vi "Actor Core.vi"(8 "error in":errorcluster, 11 "Nested in":refnum<class "ActorUITemplate.lvclass">) -> (0 "error out":errorcluster, 3 "Actor out":refnum<class "Actor.lvclass">)   [LabVIEW 2021, in "ActorUITemplate.lvclass"]
doc: "(<B>Filename</B>: Actor Framework.lvlib:Actor.lvclass:Actor Core.vi)\n\nReceives messages to the actor, reacts to them, and initiates any error handling that may shut the actor down.\n\nDescendant classes may override this VI to append parallel tasks for the actor to complete while it handles messages. Overrides use the Call Parent Method node."
uses:
  ActorUITemplate.lvclass
  C:/Program Files (x86)/National Instruments/LabVIEW 2021/user.lib/John_Lib/AbstractActorTemplate/AbstractActorTemplate/UIActorTop.lvclass
  C:/Program Files (x86)/National Instruments/LabVIEW 2021/vi.lib/ActorFramework/Actor/Actor.lvclass
  <vilib>/ActorFramework/Actor/Actor.lvclass
  TopRef.ctl
  ActorUITemplate.lvclass/ActorUITemplate.ctl
  <vilib>/ActorFramework/Actor/Actor.lvclass/Actor.ctl
  <vilib>/ActorFramework/Message Enqueuer/Message Enqueuer.lvclass/Message Enqueuer.ctl
  <vilib>/ActorFramework/Message Enqueuer/Init from Existing Queue.vi
  <vilib>/ActorFramework/Message Enqueuer/Enqueue.vi
  <vilib>/ActorFramework/Stop Msg/Stop Msg.lvclass
  C:/Program Files (x86)/National Instruments/LabVIEW 2021/vi.lib/ActorFramework/Message/Message.lvclass
  <vilib>/Utility/error.llb/Trim Whitespace.vi
  <vilib>/ActorFramework/Message Priority Queue/Priority Enqueue.vi
  <userlib>/John_Lib/OPCUA/OPCUA.lvclass
  <vilib>/ActorFramework/Message Enqueuer/Message Enqueuer.lvclass
  <userlib>/John_Lib/AbstractActorTemplate/AbstractActorTemplate/UIActorTop.lvclass
  C:/Program Files (x86)/National Instruments/LabVIEW 2021/project/Create Actor from Template/_ActorUITemplate/ActorUITemplate.lvclass
types:
  T1 = typedef "ActorUITemplate.lvclass/TopRef.ctl" = cluster{"Str Refnum":refnum<vi>}
  T2 = enum32{"Invalid", "Standard", "Closed", "Hidden", "Minimized", "Maximized"}
  T3 = enum32{"invalid app kind", "Development System", "Run Time System", "Student Edition", "Embedded LabVIEW", "Evaluation", "Custom"}
  T4 = cluster{"Core":cluster{"Current VI Reference":refnum<vi>, "Close Panel on Exit?":bool}, "Your Boolean data":bool, "Your string data":string}
  T5 = cluster{"Current VI Reference":refnum<vi>, "Close Panel on Exit?":bool}
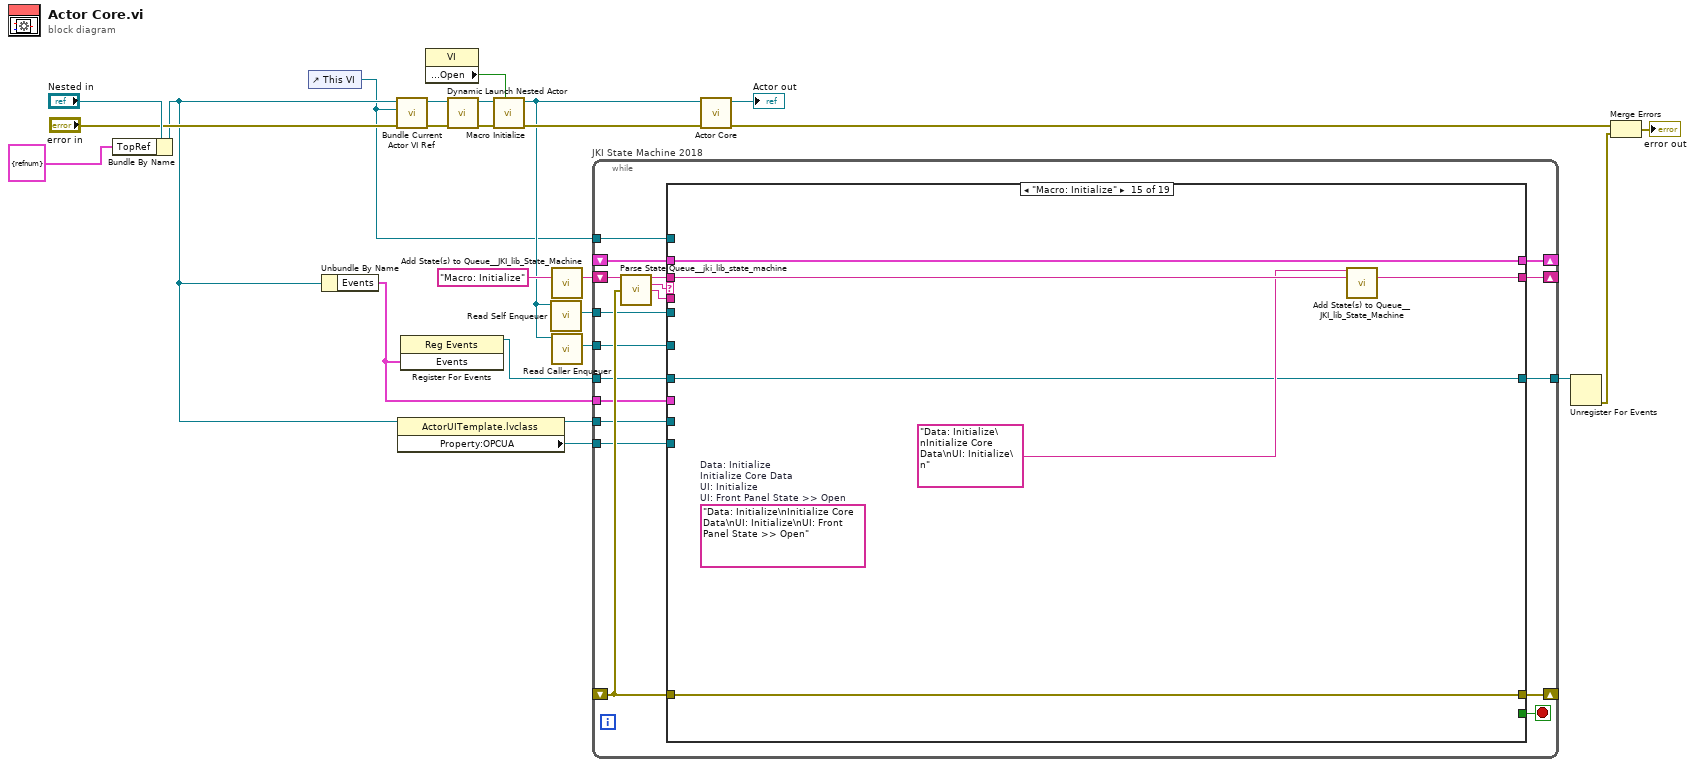
[diagram p0: block diagram]
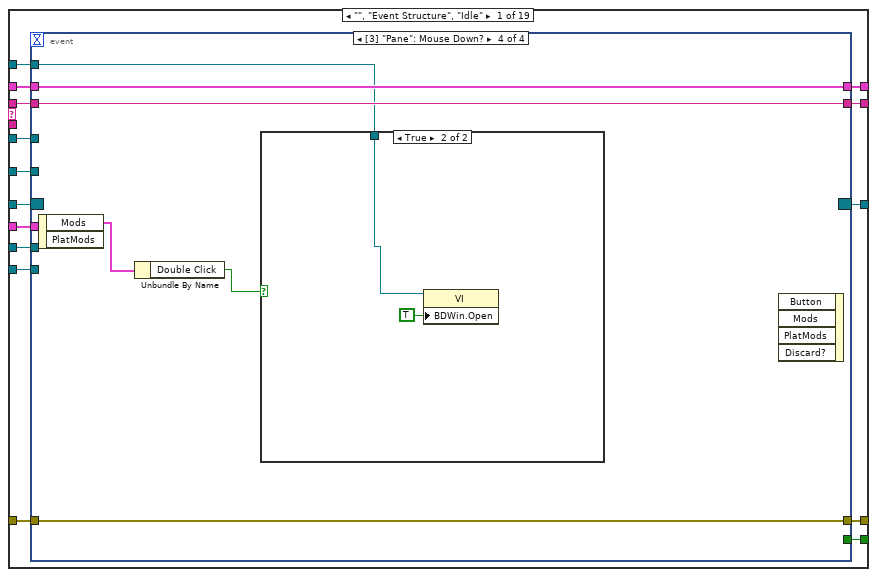
[diagram p2: hidden frame]
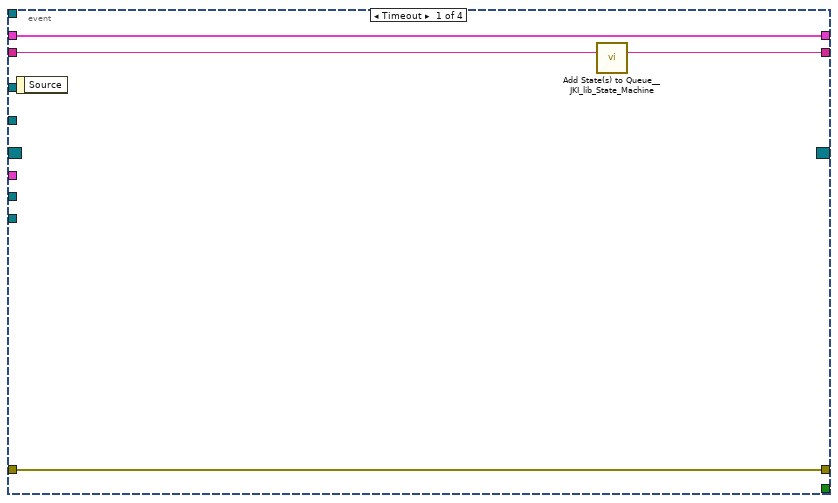
[diagram p3: hidden frame]
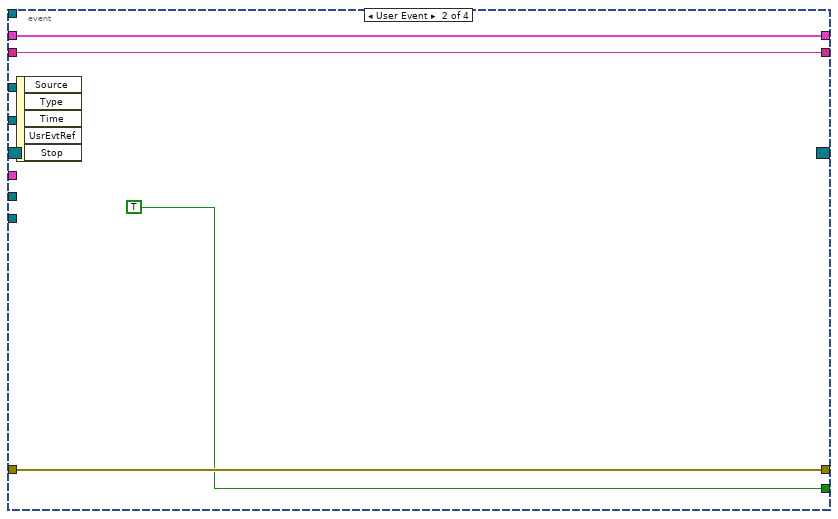
[diagram p4: hidden frame]
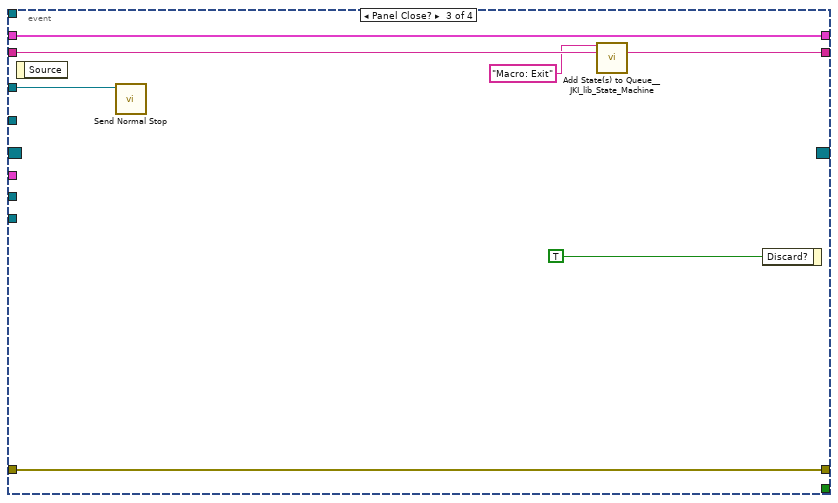
[diagram p5: hidden frame]
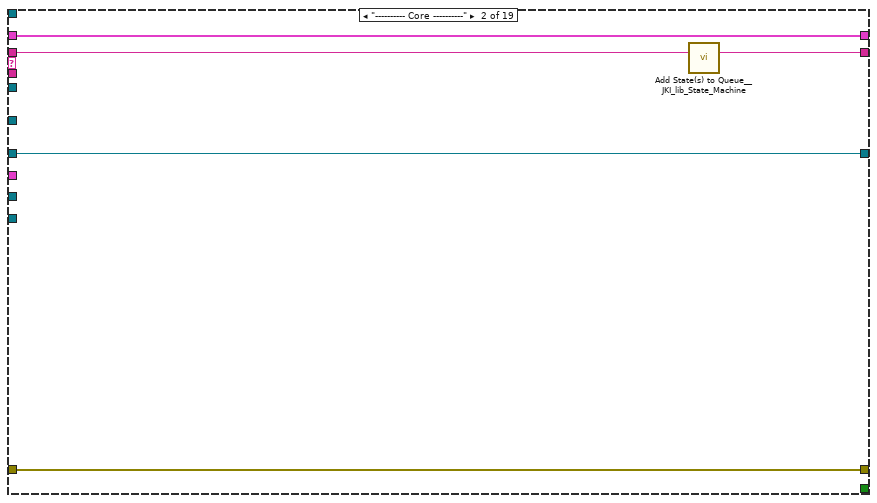
[diagram p7: hidden frame]
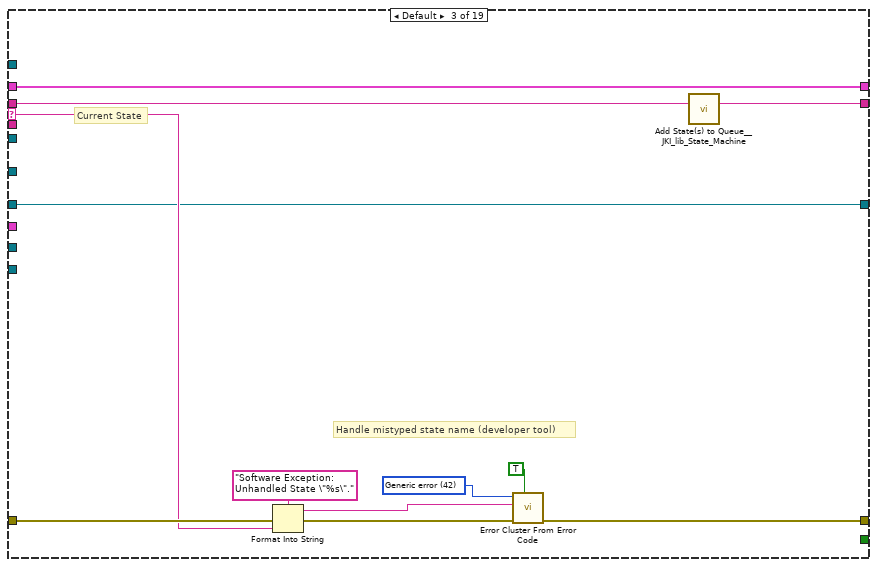
[diagram p8: hidden frame]
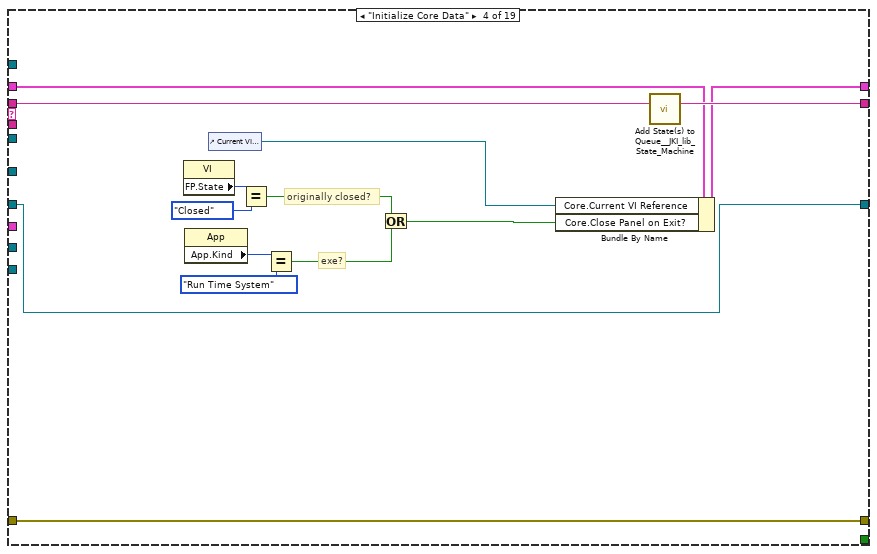
[diagram p9: hidden frame]
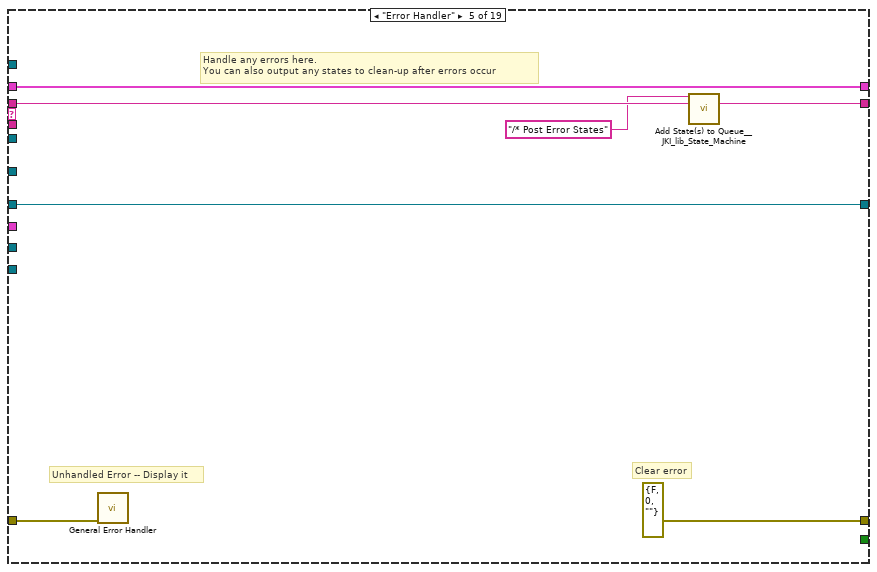
[diagram p10: hidden frame]
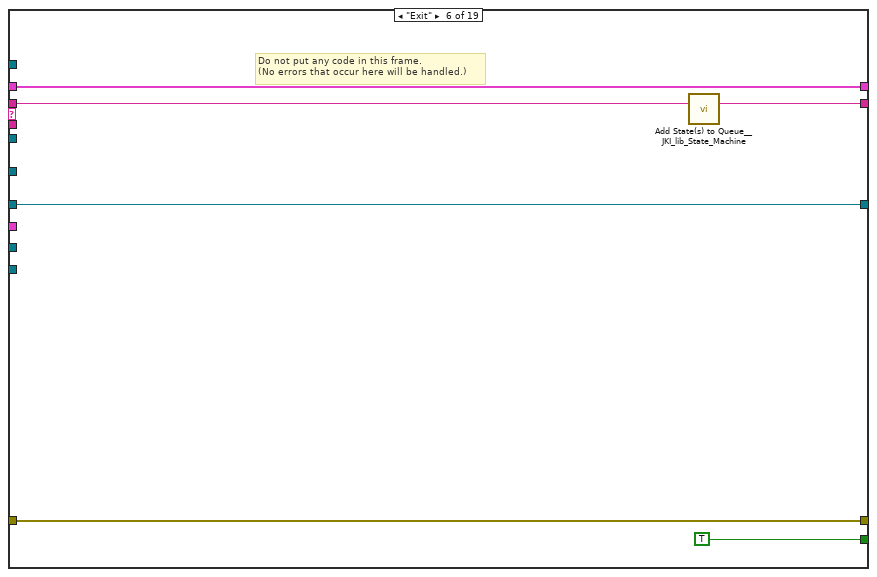
[diagram p11: hidden frame]
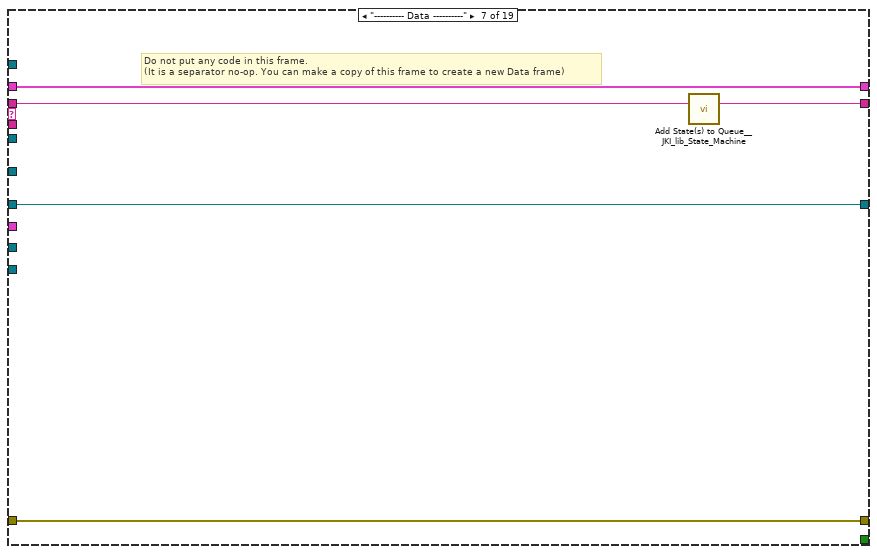
[diagram p12: hidden frame]
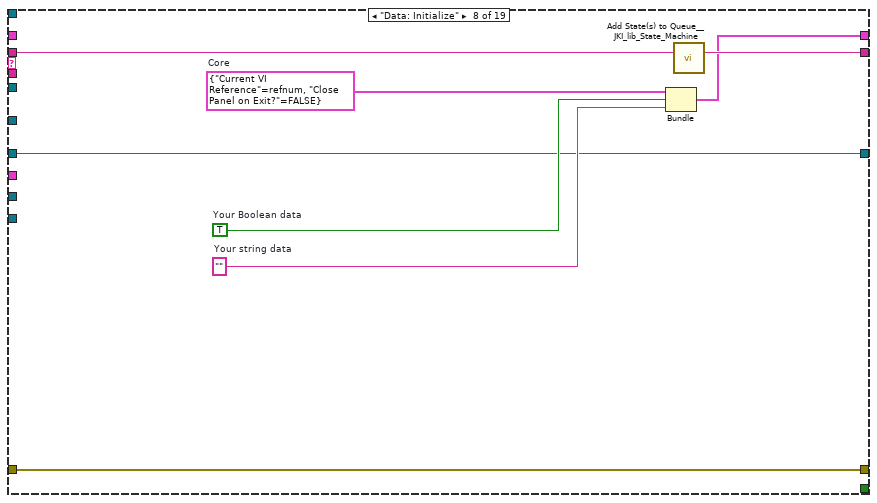
[diagram p13: hidden frame]
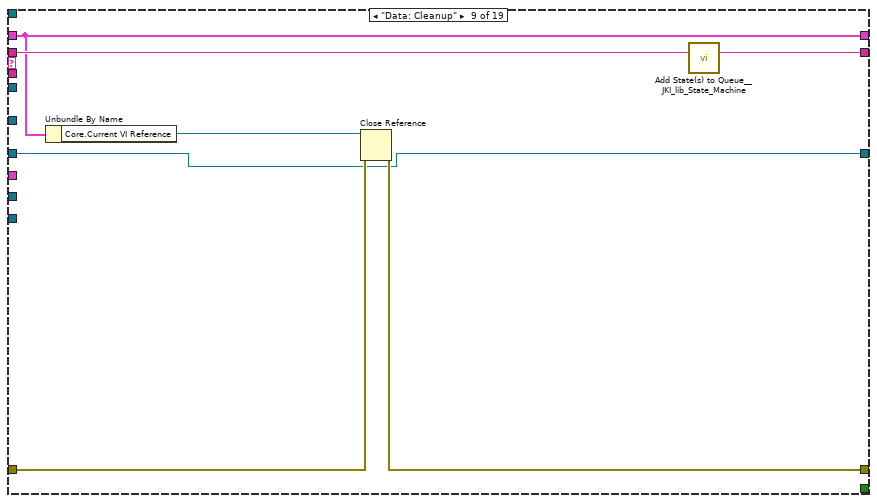
[diagram p14: hidden frame]
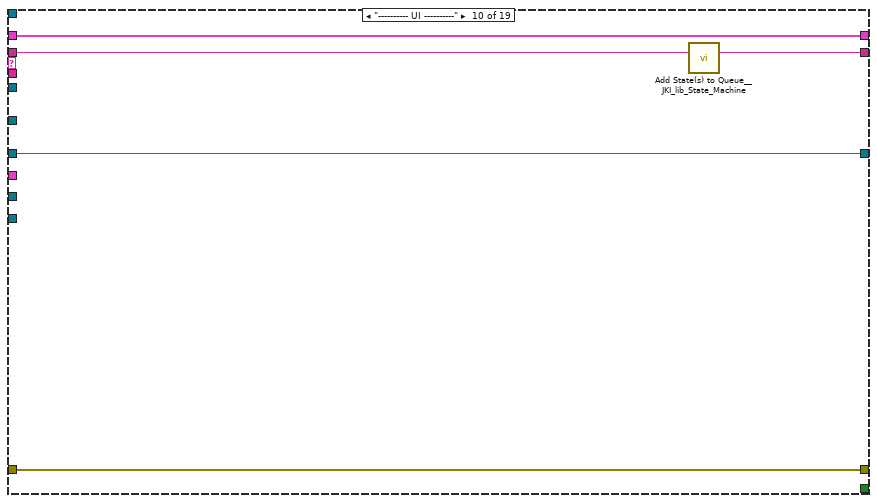
[diagram p15: hidden frame]
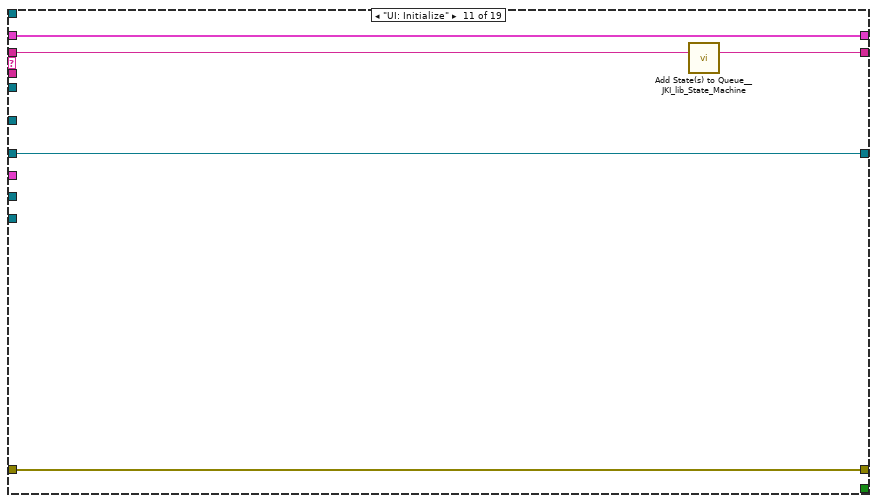
[diagram p16: hidden frame]
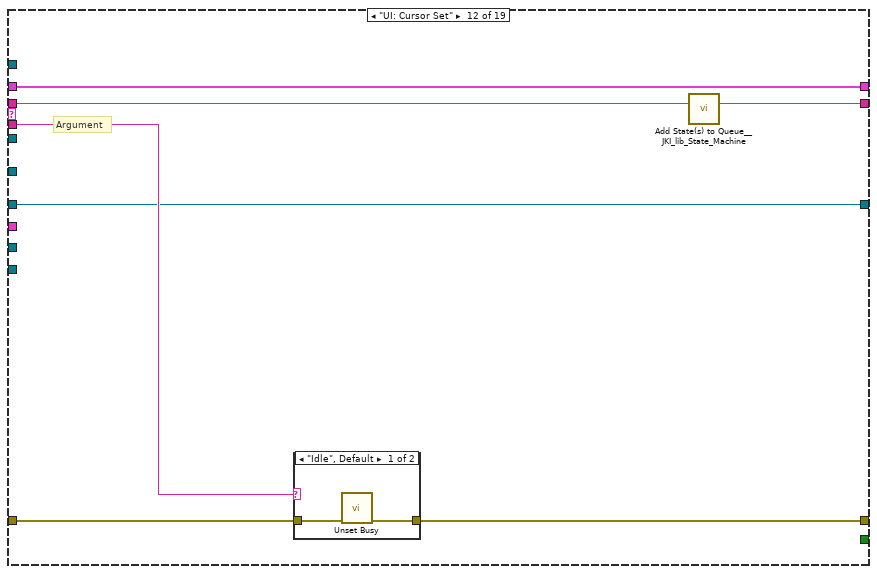
[diagram p17: hidden frame]
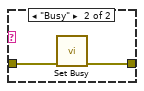
[diagram p18: hidden frame]
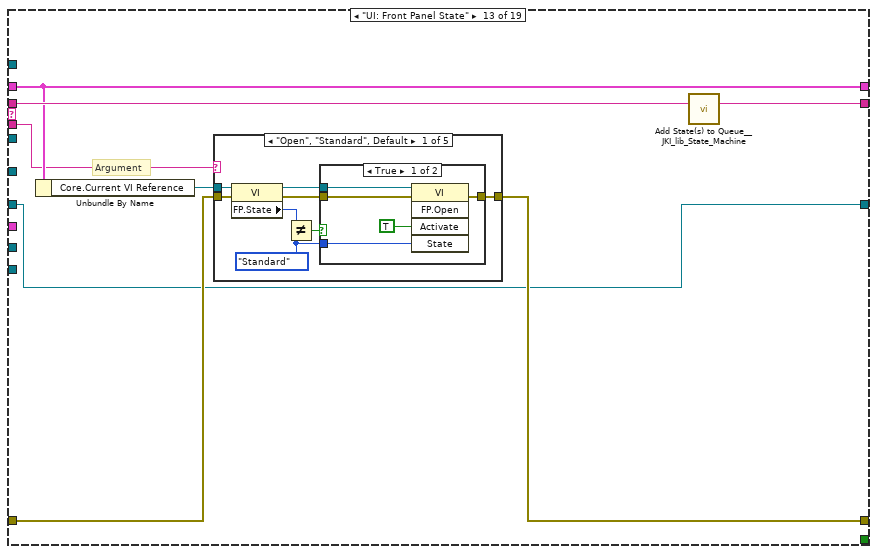
[diagram p19: hidden frame]
diagram:
  n1 = Bundle By Name(cluster="Nested in", "TopRef"=T1 {"Str Refnum"=refnum}) -> (w3:refnum<class "ActorUITemplate.lvclass">)
  n2 = control-ref of="This VI"() -> (w1:refnum<vi>)
  n3 = Unbundle By Name(w3) -> ("Events"=w10:cluster{"Stop":refnum<user-event>})
  n4 = call <userlib>:"Bundle Current Actor VI Ref.vi"("error in (no error)"="error in", "This VI"=w1, "UI ActorTop in"=w3) -> ("error out"=w15:errorcluster, "UI ActorTop out"=w16:refnum<class "ActorUITemplate.lvclass">)  [unwired: 5 in, 2 out]
  n5 = property class="ActorUITemplate.lvclass"(reference=w3) -> (reference out=w11:refnum<class "ActorUITemplate.lvclass">, "Property:OPCUA"=w12:refnum<class "OPCUA.lvclass">)  [unwired: 1 in, 1 out]
  n6 = register-events ("Main Register for Events")(w10) -> (reference out=w9:refnum<event-registration>)  [unwired: 2 in, 1 out]
  n7 = property class="VI"() -> ("Front Panel.Open"=w22:bool)  [unwired: 2 in, 2 out]
  n8 = call-dynamic "Dynamic Launch Nested Actor.vi"("error in (no error)"=w15, "UI ActorTop in"=w16) -> ("error out"=w23:errorcluster, "UI ActorTop out"=w24:refnum<class "ActorUITemplate.lvclass">)  [unwired: 8 in]
  n9 = call-dynamic "Macro Initialize.vi"("Front Panel Window:Open"=w22, "error in (no error)"=w23, "UI ActorTop in"=w24) -> ("error out"=w18:errorcluster, "UI ActorTop out"=w4:refnum<class "ActorUITemplate.lvclass">)  [unwired: 7 in]
  n10 = call <vilib>:"Read Self Enqueuer.vi"("Actor"=w4) -> ("Self Enqueuer"=w8:refnum<class "Message Enqueuer.lvclass">)  [unwired: 10 in]
  n11 = call <vilib>:"Add State(s) to Queue__JKI_lib_State_Machine.vi"("State(s) in (\"\")"="Macro: Initialize") -> ("States Out"=w5:string)  [unwired: 14 in]
  n12 = call <vilib>:"Read Caller Enqueuer.vi"("Actor"=w4) -> ("Caller Enqueuer"=w7:refnum<class "Message Enqueuer.lvclass">)  [unwired: 10 in]
  n13 = while "JKI State Machine 2018" {
    shift-right: [w36] -> _
    shift-left: _ -> [w35]
    shift-right: [w39] -> _
    shift-left: _ -> [w34]
    shift-right: [w38] -> _
    shift-left: w5 -> [w40]
    tunnel: w7 -> [w33]
    tunnel: w8 -> [w32]
    tunnel: w9 -> [w31]
    tunnel: [w30] -> w2
    tunnel: w10 -> [w29]
    tunnel: w11 -> [w28]
    tunnel: w12 -> [w27]
    tunnel: w1 -> [w26]
    stop <- w37 stop-if-true
    n14 = call <vilib>:"Parse State Queue__jki_lib_state_machine.vi"("State Queue"=w40, "Error In (no error)"=w34) -> ("Remaining States"=w42:string, "Current State"=w43:string, "Arguments"=w41:string)  [unwired: 10 in, 1 out]
    n15 = case shown="\"Macro: Initialize\"" w43 {
      selector: w43 -> [_ _ w88 _ _ _ _ _ _ _ _ _ _ _ _ _ _ _ _]
      tunnel: w42 -> [w58 w86 w92 w112 w119 w125 w130 w138 w145 w150 w155 w162 w174 w244 w250 w261 w266 w271 w276]
      tunnel: w41 -> [_ _ _ _ _ _ _ _ _ _ _ w157 w168 _ _ _ _ _ _]
      tunnel: w35 -> [w56 w83 w90 w105 w116 w123 w127 _ w140 w147 w153 w160 w170 w241 w247 w258 w263 w268 w273]
      tunnel: [w55 w84 w94 w109 errorcluster {"status"=FALSE, "code"=0, "source"=""} ("error out") w122 w128 w135 w141 w148 w152 w158 w171 w242 w248 w259 w264 w269 w274] -> w39
      tunnel: w34 -> [w54 w84 w93 w109 w115 w122 w128 w135 w142 w148 w152 w159 w172 w242 w248 w259 w264 w269 w274]
      tunnel: [w57 w85 w91 w111 w118 w124 w129 w137 w144 w149 w154 w161 w173 w243 w249 w260 w265 w270 w275] -> w38
      tunnel: [w49 _ _ _ _ TRUE _ _ _ _ _ _ _ _ _ _ _ _ _] -> w37
      tunnel: [w53 w83 w90 w110 w116 w123 w127 w136 w140 w147 w153 w160 w170 w241 w247 w258 w263 w268 w273] -> w36
      tunnel: w33 -> [w52 _ _ _ _ _ _ _ _ _ _ _ _ _ _ _ _ _ _]
      tunnel: w32 -> [w51 _ _ _ _ _ _ _ _ _ _ _ _ _ _ _ _ _ _]
      tunnel: w31 -> [w50 w82 w87 w99 w113 w120 w126 w131 w139 w146 w151 w156 w167 w240 w245 w251 w262 w267 w272]
      tunnel: [w48 w82 w87 w99 w113 w120 w126 w131 w139 w146 w151 w156 w167 w240 w245 w251 w262 w267 w272] -> w30
      tunnel: w29 -> [w47 _ _ _ _ _ _ _ _ _ _ _ _ _ _ _ _ _ _]
      tunnel: w28 -> [w46 _ _ _ _ _ _ _ _ _ _ _ _ _ _ _ _ _ _]
      tunnel: w27 -> [w45 _ _ _ _ _ _ _ _ _ _ _ _ _ _ _ _ _ _]
      tunnel: w26 -> [w44 _ _ _ _ _ _ _ _ _ _ _ _ _ _ _ _ _ _]
      frame "", "Event Structure", "Idle" {
        n16 = event shown="[3] \"Pane\": Mouse Down?" {
          selector: w50 -> [_ _ _ _]
          dyn-events: [_ _ _ _] -> w48
          timeout: _ -> [_ _ _ _]
          tunnel: w58 -> [w62 w65 w73 w79]
          tunnel: [w61 w65 w72 w79] -> w57
          tunnel: w56 -> [w59 w66 w70 w77]
          tunnel: [w60 w64 w71 w78] -> w55
          tunnel: w54 -> [w60 w64 w71 w78]
          tunnel: [w59 w66 w70 w77] -> w53
          tunnel: w52 -> [_ _ _ _]
          tunnel: w51 -> [_ _ w67 _]
          tunnel: [_ TRUE _ _] -> w49
          tunnel: w47 -> [_ _ _ _]
          tunnel: w46 -> [_ _ _ _]
          tunnel: w45 -> [_ _ _ _]
          tunnel: w44 -> [_ _ _ w74]
          event Timeout {
            n17 = event-data() -> ()  [unwired: 1 in, 1 out]
            n18 = call <vilib>:"Add State(s) to Queue__JKI_lib_State_Machine.vi"("State(s) in (\"\")"=w62) -> ("States Out"=w61:string)  [unwired: 14 in]
          }
          event User Event {
            n19 = event-data() -> ()  [unwired: 1 in, 5 out]
          }
          event Panel Close? {
            n20 = event-data() -> ()  [unwired: 1 in, 1 out]
            n21 = call <vilib>:"Send Normal Stop.vi"("Message Enqueuer"=w67) -> ()  [unwired: 10 in, 1 out]
            n22 = call <vilib>:"Add State(s) to Queue__JKI_lib_State_Machine.vi"("State(s) in Front (\"\")"="Macro: Exit", "State(s) in (\"\")"=w73) -> ("States Out"=w72:string)  [unwired: 13 in]
            n23 = event-data("Discard?"=TRUE) -> ()  [unwired: 1 in, 1 out]
          }
          event Mouse Down? {
            n24 = event-data() -> ("Mods"=w76:cluster{"Double Click":bool, "Menu Key":bool})  [unwired: 1 in, 1 out]
            n25 = Unbundle By Name(w76) -> ("Double Click"=w75:bool)
            n26 = case shown="True" w75 {
              tunnel: w74 -> [_ w81]
              frame False {
              }
              frame True {
                n27 = property class="VI"(reference=w81, "BDWin.Open"=TRUE ("Block Diagram Window:Open")) -> ()  [unwired: 1 in, 2 out]
              }
            }
            n28 = event-data() -> ()  [unwired: 5 in, 1 out]
          }
        }
      }
      frame "---------- Core ----------" {
        n29 = call <vilib>:"Add State(s) to Queue__JKI_lib_State_Machine.vi"("State(s) in (\"\")"=w86) -> ("States Out"=w85:string)  [unwired: 14 in]
      }
      frame Default {
        w97 = 42 items=["No error", "Argument error", "Memory is full", "Out of zone", "End of file", "File already open", "Generic file I/O error", "File not found", "File permission error", "Disk is full", "Duplicate path", "Too many files open", "System feature not enabled", "Resource file not found", "Cannot add resource", "Resource not found", "Image not found", "Image memory error", "Pen does not exist", "Config type invalid", "Config token not found", "Config parse error", "Config memory error", "Bad external code format", "Bad external code offset", "External code not present", "Null window", "Destroy window error", "Null menu", "Print aborted", "Bad print record", "Print driver error", "Windows error during printing", "Memory error during printing", "Print dialog error", "Generic print error", "Invalid device refnum", "Device not found", "Device parameter error", "Device unit error", "Cannot open device", "Device call aborted", "Generic error", "Cancelled by user", "Object ID too low", "Object ID too high", "Object not in heap", "Unknown heap", "Unknown object (invalid DefProc)", "Unknown object (DefProc not in table)", "Message out of range", "Invalid (null) method", "Unknown message", "Manager call not supported", "Bad address", "Network operation in progress", "Network operation timed out", "Connection is busy", "Network attribute not supported", "Network error", "Address in use", "System out of memory", "Connection aborted", "Connection refused", "Not connected", "Already connected", "Connection closed", "Initialization error (interapplication manager)", "Bad occurrence", "Wait on unbound occurrence handler", "Occurrence queue overflow", "Datalog type conflict", "Unused", "Unrecognized type (interapplication manager)", "Memory corrupt", "Failed to make temporary DLL", "Old CIN version", "Drag socket not found", "Failed to load drop-object", "Failed to register OLE object", "Failed to release OLE object", "Format specifier type mismatch", "Unknown format specifier", "Too few format specifiers", "Too many format specifiers", "Scan failed", "Newer CIN version", "Error converting to variant", "Runtime menu error", "Password tampered", "Variant attribute not found", "Incompatible variant data type", "Event data is not available", "Event Store is not present", "Occurrence is not found", "Event Queue is not created", "Event info is not available", "Refnum passed is NULL", "Error retrieving Class GUID", "Error retrieving CoClass GUID", "Error retrieving TypeLib GUID.", "Bad built application magic bytes.", "Specific driver is different from the specific driver associated with the Logical Name.", "There is no session opened to the class driver.", "Max Error", "MAX - Error with config objects", "MAX - Error loading configuration", "MAX - Group not supported"]
        # "Current State"
        # "Handle mistyped state name (developer tool)"
        n30 = Format Into String(format string="Software Exception: Unhandled State \"%s\"." ("message"), error in=w93, w88) -> (resulting string=w96:string, error out=w95:errorcluster)  [unwired: 1 in]
        n31 = call <vilib>:"Error Cluster From Error Code.vi"("show call chain? (False)"=TRUE, "error in (no error)"=w95, "error message (\"\")"=w96, "error code (0)"=w97) -> ("error out"=w94:errorcluster)  [unwired: 5 in]
        n32 = call <vilib>:"Add State(s) to Queue__JKI_lib_State_Machine.vi"("State(s) in (\"\")"=w92) -> ("States Out"=w91:string)  [unwired: 14 in]
      }
      frame "Initialize Core Data" {
        # "originally closed?"
        # "exe?"
        n33 = property class="VI"() -> ("FP.State"=w102:T2)  [unwired: 2 in, 2 out]
        n34 = property class="App"() -> ("App.Kind"=w108:T3)  [unwired: 2 in, 2 out]
        n35 = control-ref of="Current VI Reference"() -> (w103:refnum<vi>)
        n36 = Equal?(x=w102, y=T2."Closed" ("Front Panel Window:State")) -> (x = y?=w100:bool)
        n37 = Equal?(x=w108, y=T3."Run Time System" ("Application:Kind")) -> (x = y?=w106:bool)
        n38 = Or(x=w100, y=w106) -> (x .or. y?=w104:bool)
        n39 = Bundle By Name(cluster=w105, "Core.Current VI Reference"=w103, "Core.Close Panel on Exit?"=w104) -> (w110:T4)
        n40 = call <vilib>:"Add State(s) to Queue__JKI_lib_State_Machine.vi"("State(s) in (\"\")"=w112) -> ("States Out"=w111:string)  [unwired: 14 in]
      }
      frame "Error Handler" {
        # "Unhandled Error -- Display it"
        # "Handle any errors here.\nYou can also output any states to clean-up after errors occur"
        # "Clear error"
        n41 = call <vilib>:"General Error Handler.vi"("error in (no error)"=w115) -> ()  [unwired: 10 in, 5 out]
        n42 = call <vilib>:"Add State(s) to Queue__JKI_lib_State_Machine.vi"("State(s) in Front (\"\")"="/* Post Error States", "State(s) in (\"\")"=w119) -> ("States Out"=w118:string)  [unwired: 13 in]
      }
      frame "Exit" {
        # "Do not put any code in this frame.\n(No errors that occur here will be handled.)"
        n43 = call <vilib>:"Add State(s) to Queue__JKI_lib_State_Machine.vi"("State(s) in (\"\")"=w125) -> ("States Out"=w124:string)  [unwired: 14 in]
      }
      frame "---------- Data ----------" {
        # "Do not put any code in this frame.\n(It is a separator no-op. You can make a copy of this frame to create a new Data frame)"
        n44 = call <vilib>:"Add State(s) to Queue__JKI_lib_State_Machine.vi"("State(s) in (\"\")"=w130) -> ("States Out"=w129:string)  [unwired: 14 in]
      }
      frame "Data: Initialize" {
        w132 = T5 {"Current VI Reference"=refnum, "Close Panel on Exit?"=FALSE}  # Core
        w134 = TRUE  # Your Boolean data
        w133 = ""  # Your string data
        n45 = Bundle("Core"=w132, "Your Boolean data"=w134, "Your string data"=w133) -> (w136:T4)  [unwired: 1 in]
        n46 = call <vilib>:"Add State(s) to Queue__JKI_lib_State_Machine.vi"("State(s) in (\"\")"=w138) -> ("States Out"=w137:string)  [unwired: 14 in]
      }
      frame "Data: Cleanup" {
        n47 = Unbundle By Name(w140) -> ("Core.Current VI Reference"=w143:refnum<vi>)
        n48 = Close Reference(reference=w143, error in (no error)=w142) -> (error out=w141:errorcluster)
        n49 = call <vilib>:"Add State(s) to Queue__JKI_lib_State_Machine.vi"("State(s) in (\"\")"=w145) -> ("States Out"=w144:string)  [unwired: 14 in]
      }
      frame "---------- UI ----------" {
        n50 = call <vilib>:"Add State(s) to Queue__JKI_lib_State_Machine.vi"("State(s) in (\"\")"=w150) -> ("States Out"=w149:string)  [unwired: 14 in]
      }
      frame "UI: Initialize" {
        n51 = call <vilib>:"Add State(s) to Queue__JKI_lib_State_Machine.vi"("State(s) in (\"\")"=w155) -> ("States Out"=w154:string)  [unwired: 14 in]
      }
      frame "UI: Cursor Set" {
        # "Argument"
        n52 = case shown="\"Idle\", Default" w157 {
          tunnel: w159 -> [w164 w166]
          tunnel: [w163 w165] -> w158
          frame "Idle", Default {
            n53 = call <vilib>:"Unset Busy.vi"("error in (no error)"=w164) -> ("error out"=w163:errorcluster)  [unwired: 10 in]
          }
          frame "Busy" {
            n54 = call <vilib>:"Set Busy.vi"("error in (no error)"=w166) -> ("error out"=w165:errorcluster)  [unwired: 9 in, 1 out]
          }
        }
        n55 = call <vilib>:"Add State(s) to Queue__JKI_lib_State_Machine.vi"("State(s) in (\"\")"=w162) -> ("States Out"=w161:string)  [unwired: 14 in]
      }
      frame "UI: Front Panel State" {
        # "Argument"
        n56 = Unbundle By Name(w170) -> ("Core.Current VI Reference"=w169:refnum<vi>)
        n57 = case shown="\"Open\", \"Standard\", Default" w168 {
          tunnel: w172 -> [w180 w195 w206 w219 w232]
          tunnel: [w182 w196 w208 w221 w234] -> w171
          tunnel: w169 -> [w181 w193 w207 w220 w233]
          frame "Open", "Standard", Default {
            w175 = T2."Standard" ("State")
            n58 = property class="VI"(reference=w181, error in=w180) -> (reference out=w178:refnum<vi>, error out=w179:errorcluster, "FP.State"=w177:T2)
            n59 = Not Equal?(x=w177, y=w175) -> (x != y?=w176:bool)
            n60 = case shown="True" w176 {
              tunnel: [w186 w188] -> w182
              tunnel: w179 -> [w185 w188]
              tunnel: w178 -> [w184 _]
              tunnel: w175 -> [w183 _]
              frame True {
                n61 = invoke class="VI" method="FP.Open"(reference=w184, error in=w185, "Activate"=TRUE, "State"=w183) -> (error out=w186:errorcluster)  [unwired: 1 in, 4 out]
              }
              frame False {
              }
            }
          }
          frame "Close", "Closed" {
            n62 = property class="VI"(reference=w193, error in=w195) -> (reference out=w192:refnum<vi>, error out=w194:errorcluster, "FP.State"=w190:T2)
            n63 = Not Equal?(x=w190, y=T2."Closed" ("Front Panel Window:State")) -> (x != y?=w189:bool)
            n64 = case shown="True" w189 {
              tunnel: [w197 w200] -> w196
              tunnel: w194 -> [w197 w199]
              tunnel: w192 -> [_ w198]
              frame False {
              }
              frame True {
                n65 = invoke class="VI" method="FP.Close"(reference=w198, error in=w199) -> (error out=w200:errorcluster)  [unwired: 1 in, 2 out]
              }
            }
          }
          frame "Hidden", "Hide" {
            w201 = T2."Hidden" ("State")
            n66 = property class="VI"(reference=w207, error in=w206) -> (reference out=w204:refnum<vi>, error out=w205:errorcluster, "FP.State"=w203:T2)
            n67 = Not Equal?(x=w203, y=w201) -> (x != y?=w202:bool)
            n68 = case shown="True" w202 {
              tunnel: [w212 w213] -> w208
              tunnel: w205 -> [w211 w213]
              tunnel: w204 -> [w210 _]
              tunnel: w201 -> [w209 _]
              frame True {
                n69 = invoke class="VI" method="FP.Open"(reference=w210, error in=w211, "State"=w209) -> (error out=w212:errorcluster)  [unwired: 2 in, 4 out]
              }
              frame False {
              }
            }
          }
          frame "Minimize", "Minimized" {
            w214 = T2."Minimized" ("State")
            n70 = property class="VI"(reference=w220, error in=w219) -> (reference out=w217:refnum<vi>, error out=w218:errorcluster, "FP.State"=w216:T2)
            n71 = Not Equal?(x=w216, y=w214) -> (x != y?=w215:bool)
            n72 = case shown="True" w215 {
              tunnel: [w225 w226] -> w221
              tunnel: w218 -> [w224 w226]
              tunnel: w217 -> [w223 _]
              tunnel: w214 -> [w222 _]
              frame True {
                n73 = invoke class="VI" method="FP.Open"(reference=w223, error in=w224, "State"=w222) -> (error out=w225:errorcluster)  [unwired: 2 in, 4 out]
              }
              frame False {
              }
            }
          }
          frame "Maximize", "Maximized" {
            w227 = T2."Maximized" ("State")
            n74 = property class="VI"(reference=w233, error in=w232) -> (reference out=w230:refnum<vi>, error out=w231:errorcluster, "FP.State"=w229:T2)
            n75 = Not Equal?(x=w229, y=w227) -> (x != y?=w228:bool)
            n76 = case shown="True" w228 {
              tunnel: [w238 w239] -> w234
              tunnel: w231 -> [w237 w239]
              tunnel: w230 -> [w236 _]
              tunnel: w227 -> [w235 _]
              frame True {
                n77 = invoke class="VI" method="FP.Open"(reference=w236, error in=w237, "State"=w235) -> (error out=w238:errorcluster)  [unwired: 2 in, 4 out]
              }
              frame False {
              }
            }
          }
        }
        n78 = call <vilib>:"Add State(s) to Queue__JKI_lib_State_Machine.vi"("State(s) in (\"\")"=w174) -> ("States Out"=w173:string)  [unwired: 14 in]
      }
      frame "---------- Macro ----------" {
        n79 = call <vilib>:"Add State(s) to Queue__JKI_lib_State_Machine.vi"("State(s) in (\"\")"=w244) -> ("States Out"=w243:string)  [unwired: 14 in]
      }
      frame "Macro: Initialize" {
        (unwired) "Data: Initialize\nInitialize Core Data\nUI: Initialize\nUI: Front Panel State >> Open"  # Data: Initialize Initialize Core Data UI: Initialize UI: Front Panel State >> Open
        n80 = call <vilib>:"Add State(s) to Queue__JKI_lib_State_Machine.vi"("State(s) in Front (\"\")"="Data: Initialize\nInitialize Core Data\nUI: Initialize\n", "State(s) in (\"\")"=w250) -> ("States Out"=w249:string)  [unwired: 13 in]
      }
      frame "Macro: Exit" {
        n81 = Unbundle By Name(w258) -> ("Core.Close Panel on Exit?"=w257:bool)
        n82 = Select(t="UI: Front Panel State >> Close", s=w257, f="") -> (s? t:f=w254:string)
        n83 = call <vilib>:"Add State(s) to Queue__JKI_lib_State_Machine.vi"("State(s) in (\"\")"=w254, "State(s) at Back (\"\")"="Data: Cleanup\nExit") -> ("States Out"=w252:string)  [unwired: 13 in]
        n84 = call <vilib>:"Add State(s) to Queue__JKI_lib_State_Machine.vi"("State(s) in Front (\"\")"=w252, "State(s) in (\"\")"=w261) -> ("States Out"=w260:string)  [unwired: 13 in]
      }
      frame "---------- New Category ----------" {
        n85 = call <vilib>:"Add State(s) to Queue__JKI_lib_State_Machine.vi"("State(s) in (\"\")"=w266) -> ("States Out"=w265:string)  [unwired: 14 in]
      }
      frame "New Category: 1" {
        n86 = call <vilib>:"Add State(s) to Queue__JKI_lib_State_Machine.vi"("State(s) in (\"\")"=w271) -> ("States Out"=w270:string)  [unwired: 14 in]
      }
      frame "New Category: 2" {
        n87 = call <vilib>:"Add State(s) to Queue__JKI_lib_State_Machine.vi"("State(s) in (\"\")"=w276) -> ("States Out"=w275:string)  [unwired: 14 in]
      }
    }
  }
  n88 = call-parent "Actor Core.vi"("error in"=w18, "Actor in"=w4) -> ("error out"=w20:errorcluster, "Actor out"=→"Actor out":refnum<class "Actor.lvclass">)  [unwired: 8 in]
  n89 = Unregister For Events(event registration refnum=w2) -> (error out=w21:errorcluster)  [unwired: 1 in]
  n90 = Merge Errors(w20, w21) -> (→"error out":errorcluster)
